vi "PC motor control demo.vi"() -> ()   [LabVIEW 2012]
uses:
  <vilib>/Utility/inputDevices.llb/closeKeyboard.vi
  <vilib>/Utility/inputDevices.llb/keyboardAcquire.vi
panel:
  out "Port\nRudder":i32
  out "Right\nRubber":i32
  in  "Balance Rudders":i32(slide) scale=-200.0..200.0
  out "Port\nMotor":i32
  out "Starboard\nMotor":i32
  in  "Balance motors":i32(slide) scale=-200.0..200.0
  out "Rudders Direction":i32(knob) scale=500.0..2500.0
  out "Motors Speed":i32(knob) scale=500.0..2500.0
  in  "stop":bool
  # "Move the arrow keys to change the motor speed and rudder"
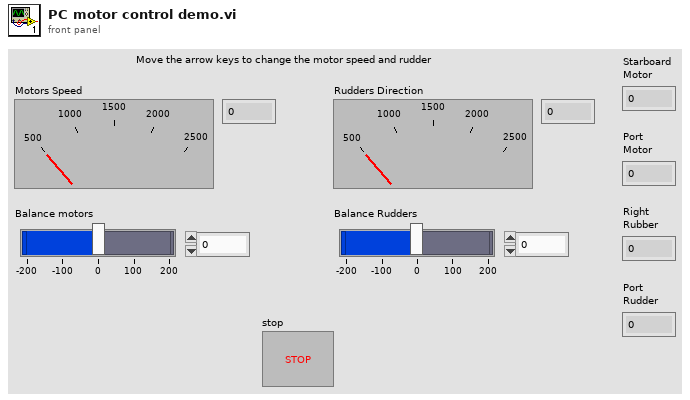
[diagram p1: front panel]
types:
  T1 = enum16{"0", "1", "2", "3", "4", "5", "6", "7", "8", "9", "A", "B", "C", "D", "E", "F", "G", "H", "I", "J", "K", "L", "M", "N", "O", "P", "Q", "R", "S", "T", "U", "V", "W", "X", "Y", "Z", "F1", "F2", "F3", "F4", "F5", "F6", "F7", "F8", "F9", "F10", "F11", "F12", "F13", "F14", "F15", "ADD", "BACK", "BACKSLASH", "CAPITAL", "COMMA", "DECIMAL", "DELETE", "DIVIDE", "DOWN", "END", "EQUALS", "ESCAPE", "GRAVE (`)", "HOME", "INSERT", "LBRACKET", "LCONTROL", "LEFT", "L ALT", "LSHIFT", "LWIN", "MINUS", "MULTIPLY", "NEXT", "NUMLOCK", "NUMPAD_0", "NUMPAD_1", "NUMPAD_2", "NUMPAD_3", "NUMPAD_4", "NUMPAD_5", "NUMPAD_6", "NUMPAD_7", "NUMPAD_8", "NUMPAD_9", "PAUSE", "PERIOD", "PRIOR (PG UP)", "RBRACKET", "RCONTROL", "RETURN", "RIGHT", "R ALT", "RSHIFT", "RWIN", "SCROLL", "SEMICOLON", "SLASH", "SPACE", "SUBTRACT", "TAB", "UP", "ENTER (num pad)", "' (quote)"}[]
  T2 = enum16{"0", "1", "2", "3", "4", "5", "6", "7", "8", "9", "A", "B", "C", "D", "E", "F", "G", "H", "I", "J", "K", "L", "M", "N", "O", "P", "Q", "R", "S", "T", "U", "V", "W", "X", "Y", "Z", "F1", "F2", "F3", "F4", "F5", "F6", "F7", "F8", "F9", "F10", "F11", "F12", "F13", "F14", "F15", "ADD", "BACK", "BACKSLASH", "CAPITAL", "COMMA", "DECIMAL", "DELETE", "DIVIDE", "DOWN", "END", "EQUALS", "ESCAPE", "GRAVE (`)", "HOME", "INSERT", "LBRACKET", "LCONTROL", "LEFT", "L ALT", "LSHIFT", "LWIN", "MINUS", "MULTIPLY", "NEXT", "NUMLOCK", "NUMPAD_0", "NUMPAD_1", "NUMPAD_2", "NUMPAD_3", "NUMPAD_4", "NUMPAD_5", "NUMPAD_6", "NUMPAD_7", "NUMPAD_8", "NUMPAD_9", "PAUSE", "PERIOD", "PRIOR (PG UP)", "RBRACKET", "RCONTROL", "RETURN", "RIGHT", "R ALT", "RSHIFT", "RWIN", "SCROLL", "SEMICOLON", "SLASH", "SPACE", "SUBTRACT", "TAB", "UP", "ENTER (num pad)", "' (quote)"}
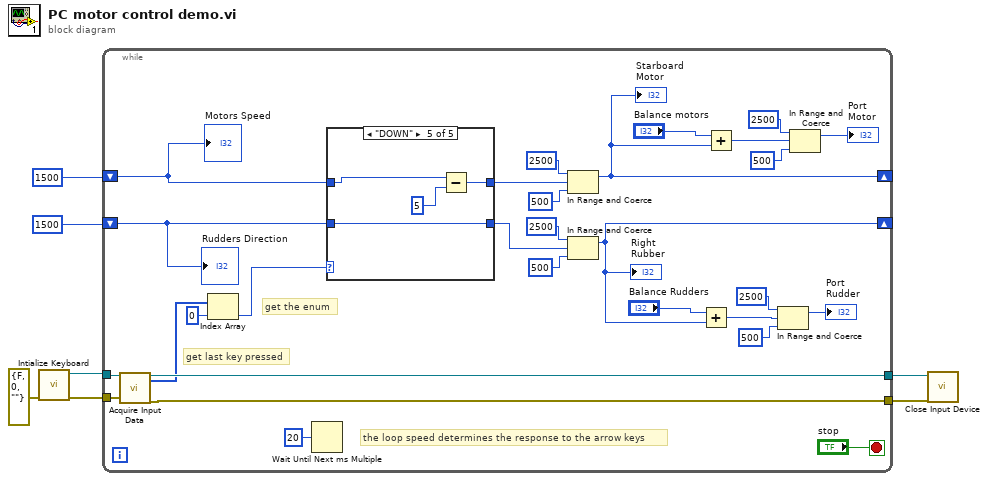
[diagram p0: block diagram]
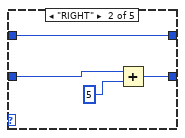
[diagram p3: hidden frame]
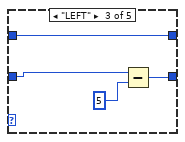
[diagram p4: hidden frame]
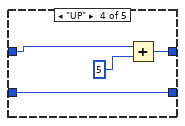
[diagram p5: hidden frame]
diagram:
  n1 = call <vilib>:"Intialize Keyboard.vi"("error in (no error)"=errorcluster {"status"=FALSE, "code"=0, "source"=""}) -> ("error out"=w7:errorcluster, "device ID"=w5:refnum<k1>)  [unwired: 9 in]
  n2 = while {
    tunnel: w7 -> [w35]
    tunnel: w5 -> [w34]
    tunnel: [w33] -> w4
    tunnel: [w32] -> w3
    shift-right: [w18] -> _
    shift-left: 1500 -> [w27]
    shift-right: [w16] -> _
    shift-left: 1500 -> [w26]
    stop <- "stop" stop-if-true
    # "get the enum"
    # "the loop speed determines the response to the arrow keys"
    # "get last key pressed"
    n3 = call-poly <vilib>:"Acquire Input Data.vi"("device ID"=w34, "error in (no error)"=w35) -> ("device ID"=w32:refnum<k1>, "keys pressed"=w31:T1, "error out"=w33:errorcluster)  [unwired: 15 in]
    n4 = Index Array(array=w31, index=0) -> (element=w29:T2)
    n5 = Wait Until Next ms Multiple(millisecond multiple=u32 20) -> ()  [unwired: 1 out]
    n6 = case shown="\"DOWN\"" w29 {
      tunnel: w27 -> [w38 w42 w46 w47 w51]
      tunnel: [w38 w42 w46 w48 w52] -> w25
      tunnel: w26 -> [w37 w40 w43 w50 w54]
      tunnel: [w37 w39 w44 w50 w54] -> w20
      frame "0", Default {
        # "use arrow\nkeys only"
      }
      frame "RIGHT" {
        n7 = Add(x=w40, y=5) -> (x+y=w39:i32)
      }
      frame "LEFT" {
        n8 = Subtract(x=w43, y=5) -> (x-y=w44:i32)
      }
      frame "UP" {
        n9 = Add(x=w47, y=5) -> (x+y=w48:i32)
      }
      frame "DOWN" {
        n10 = Subtract(x=w51, y=5) -> (x-y=w52:i32)
      }
    }
    n11 = In Range and Coerce(upper limit=2500, x=w25, lower limit=500) -> (coerced(x)=w18:i32)  [unwired: 1 out]
    "Starboard\nMotor" <- w18
    n12 = In Range and Coerce(upper limit=2500, x=w20, lower limit=500) -> (coerced(x)=w16:i32)  [unwired: 1 out]
    "Right\nRubber" <- w16
    n13 = Add(x="Balance Rudders", y=w16) -> (x+y=w9:i32)
    n14 = Add(x="Balance motors", y=w18) -> (x+y=w13:i32)
    n15 = In Range and Coerce(upper limit=2500, x=w9, lower limit=500) -> (coerced(x)=→"Port\nRudder":i32)  [unwired: 1 out]
    n16 = In Range and Coerce(upper limit=2500, x=w13, lower limit=500) -> (coerced(x)=→"Port\nMotor":i32)  [unwired: 1 out]
    "Motors Speed" <- w27
    "Rudders Direction" <- w26
  }
  n17 = call-poly <vilib>:"Close Input Device.vi"("error in (no error)"=w4, "device ID"=w3) -> ()  [unwired: 8 in, 1 out]
